vi "check_forward_scan.vi"(8 "Last Element":bool, 11 "Input":u64) -> (2 "Output Ch1":u32)   [LabVIEW 2012]
panel:
  out "Output Ch2":u32
  out "Forward?":bool
  out "New Element":bool
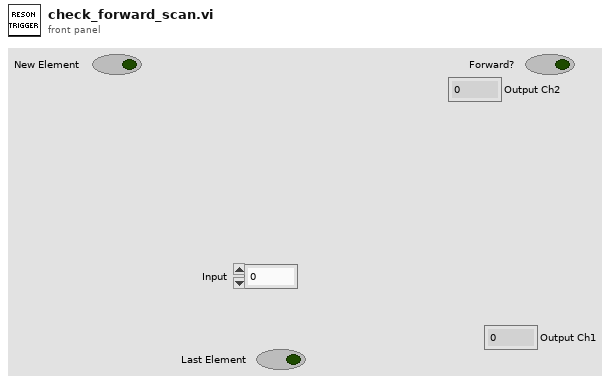
[diagram p1: front panel]
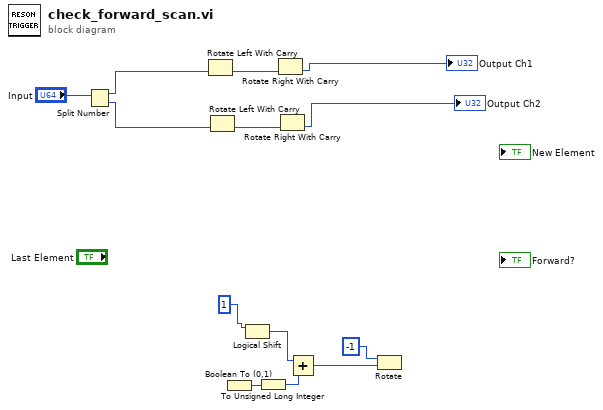
[diagram p0: block diagram]
diagram:
  n1 = Split Number(x="Input") -> (hi(x)=w3:u32, lo(x)=w6:u32)
  n2 = Rotate Left With Carry(2:w3) -> (0:w2:u32)  [unwired: 1 in, 1 out]
  n3 = Rotate Left With Carry(2:w6) -> (0:w5:u32)  [unwired: 1 in, 1 out]
  n4 = Boolean To (0,1)() -> (0, 1=w9:i16)  [unwired: 1 in]
  n5 = Logical Shift(y=i16 1) -> (x << y=w10:i16)  [unwired: 1 in]
  n6 = To Unsigned Long Integer(number=w9) -> (unsigned 32bit integer=w8:u32)
  n7 = Rotate Right With Carry(2:w2) -> (0:→"Output Ch1":u32)  [unwired: 1 in, 1 out]
  n8 = Rotate Right With Carry(2:w5) -> (0:→"Output Ch2":u32)  [unwired: 1 in, 1 out]
  n9 = Add(x=w10, y=w8) -> (x+y=w12:u32)
  n10 = Rotate(1:w12, 2:i16 -1) -> ()  [unwired: 1 out]
